vi "TAT_PLC_Data_read_BOLLEAN_I_O_SCREEN.vi"(7 "Enum":enum16{"Read", "Write"}(ring), 8 "error in (no error)":errorcluster, 10 "Array":bool[](array[boolean])) -> (0 "error out":errorcluster, 2 "Array 2":bool[](array[boolean]))   [LabVIEW 2017]
panel:
  # "INPUTS\t\t\nSR.NO\tPLC INPUT\tDESCRIPTION\tTO SOFTWARE MEMORY BIT\t\n1\tX0\tCYCLE START TOUCH BUTTON\tM0\t8192\n2\tX1\tCYCLE START TOUCH BUTTON\tM1\t8193\n3\tX2\tEMG STOP\tM2\t8194\n4\tX3\tRESET PB\tM3\t8195\n5\tX4\tPRESSURE SWITCH\tM4\t8196\n6\tX5\tSAFETY SENSOR\tM5\t8197\n7\tX6\tDOOR 1 \tM6\t8198\n8\tX7\tDOOR 2\tM7\t8199\n9\tX10\tSPARE\tM10\t8202\n10\tX11\tSHUTTLE OPEN CHECK SENSOR-X300\tM11\t8203\n11\tX12\tTHREAD LOCKER CYL COMPLETE\tM12\t8204\n12\tX13\tPUSHER HM RS\tM13\t8205\n13\tX14\tPUSHER END RS\tM14\t8206\n14\tX15\tUP DOWN CYL  HM RS\tM15\t8207\n15\tX16\tUP DOWN CYL END RS\tM16\t8208\n16\tX17\tPART CLAMP END RS\tM17\t8209\n17\tX20\t\tM20\t8212\n18\tX21\t\tM21\t8213\n19\tX22\t\tM22\t8214\n20\tX23\t\tM23\t8215\n21\tX24\t\tM24\t8216\n22\tX25\t\tM25\t8217\n\t\t\t\t\n\t\t\t\t\n\t\t\t\t\n\t\t\t\t\n\t\tOUTPUTS\t\t\nSR.NO\tPLC OUTPUT\tDESCRIPTION\tTO SOFTWARE MEMORY BIT\t\n1\tY0\tGREEN LAMP\tM30\t8222\n2\tY1\tRED LAMP\tM31\t8223\n3\tY2\tBUZZER\tM32\t8224\n4\tY3\tPART CLAMP SOL\tM33\t8225\n5\tY4\tTHREAD LOCKER ON\tM34\t8226\n6\tY5\tTHREAD LOCKER OFF\tM35\t8227\n7\tY6\tPUSHER FWD SOL\tM36\t8228\n8\tY7\tPUSHER REV SOL\tM37\t8229\n9\tY10\tUP DN CYL FWD SOL\tM38\t8230\n10\tY11\tUP DN CYL REV SOL\tM39\t8231\n11\tY12\t\tM40\t8232\n12\tY13\t\tM41\t8233\n13\tY14\t\tM42\t8234\n14\tY15\t\tM43\t8235\n15\tY16\t\tM44\t8236\n16\tY17\t\tM45\t8237\n17\tY20\t\tM46\t8238\n18\tY21\t\tM47\t8239"
  # "STATION 1\nand\nSTATION 2"
  # "CONTROL PROCESS TO  LABVIEW from PLC"
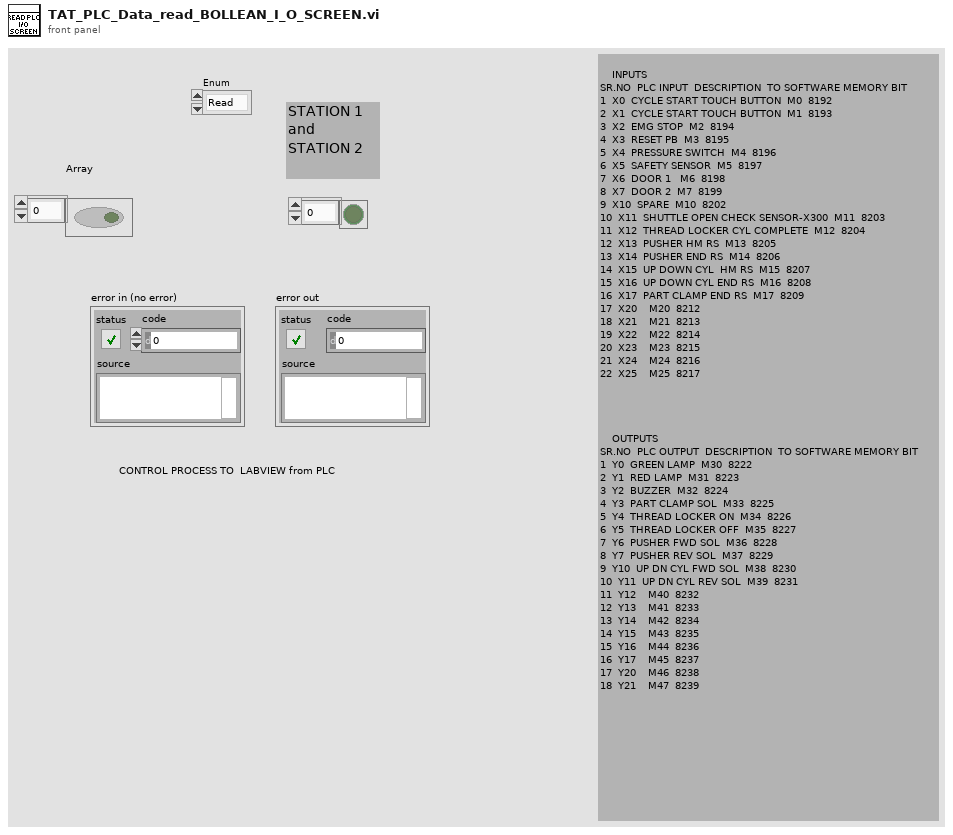
[diagram p1: front panel]
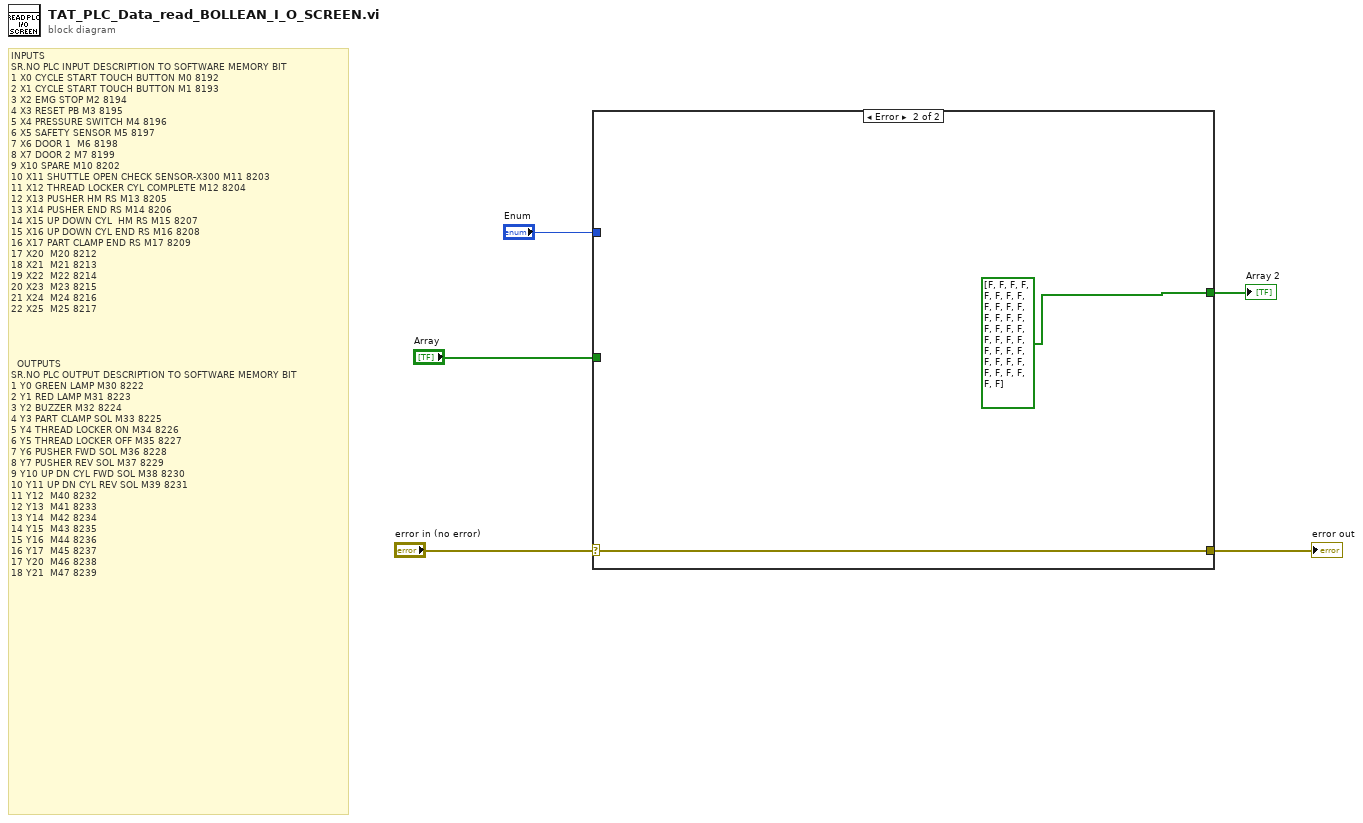
[diagram p0: block diagram]
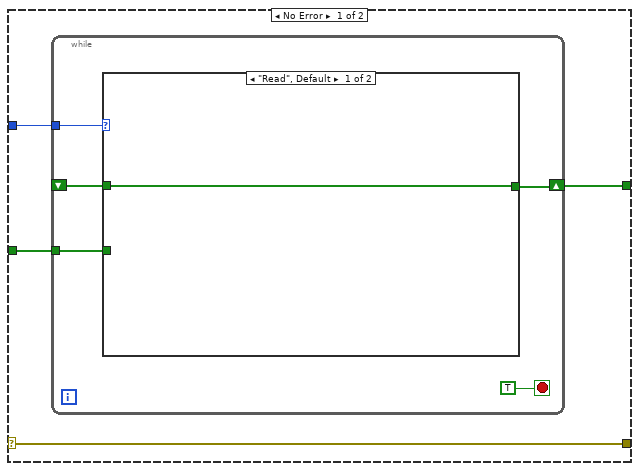
[diagram p2: hidden frame]
diagram:
  # "INPUTS\t\t\nSR.NO\tPLC INPUT\tDESCRIPTION\tTO SOFTWARE MEMORY BIT\t\n1\tX0\tCYCLE START TOUCH BUTTON\tM0\t8192\n2\tX1\tCYCLE START TOUCH BUTTON\tM1\t8193\n3\tX2\tEMG STOP\tM2\t8194\n4\tX3\tRESET PB\tM3\t8195\n5\tX4\tPRESSURE SWITCH\tM4\t8196\n6\tX5\tSAFETY SENSOR\tM5\t8197\n7\tX6\tDOOR 1 \tM6\t8198\n8\tX7\tDOOR 2\tM7\t8199\n9\tX10\tSPARE\tM10\t8202\n10\tX11\tSHUTTLE OPEN CHECK SENSOR-X300\tM11\t8203\n11\tX12\tTHREAD LOCKER CYL COMPLETE\tM12\t8204\n12\tX13\tPUSHER HM RS\tM13\t8205\n13\tX14\tPUSHER END RS\tM14\t8206\n14\tX15\tUP DOWN CYL  HM RS\tM15\t8207\n15\tX16\tUP DOWN CYL END RS\tM16\t8208\n16\tX17\tPART CLAMP END RS\tM17\t8209\n17\tX20\t\tM20\t8212\n18\tX21\t\tM21\t8213\n19\tX22\t\tM22\t8214\n20\tX23\t\tM23\t8215\n21\tX24\t\tM24\t8216\n22\tX25\t\tM25\t8217\n\t\t\t\t\n\t\t\t\t\n\t\t\t\t\n\t\t\t\t\n\t\tOUTPUTS\t\t\nSR.NO\tPLC OUTPUT\tDESCRIPTION\tTO SOFTWARE MEMORY BIT\t\n1\tY0\tGREEN LAMP\tM30\t8222\n2\tY1\tRED LAMP\tM31\t8223\n3\tY2\tBUZZER\tM32\t8224\n4\tY3\tPART CLAMP SOL\tM33\t8225\n5\tY4\tTHREAD LOCKER ON\tM34\t8226\n6\tY5\tTHREAD LOCKER OFF\tM35\t8227\n7\tY6\tPUSHER FWD SOL\tM36\t8228\n8\tY7\tPUSHER REV SOL\tM37\t8229\n9\tY10\tUP DN CYL FWD SOL\tM38\t8230\n10\tY11\tUP DN CYL REV SOL\tM39\t8231\n11\tY12\t\tM40\t8232\n12\tY13\t\tM41\t8233\n13\tY14\t\tM42\t8234\n14\tY15\t\tM43\t8235\n15\tY16\t\tM44\t8236\n16\tY17\t\tM45\t8237\n17\tY20\t\tM46\t8238\n18\tY21\t\tM47\t8239"
  n1 = case shown="Error" "error in (no error)" {
    selector: "error in (no error)" -> [w6 w18]
    tunnel: [w6 w18] -> w5
    tunnel: "Enum" -> [w9 _]
    tunnel: "Array" -> [w8 _]
    tunnel: [w7 bool[] [FALSE, FALSE, FALSE, FALSE, FALSE, FALSE, FALSE, FALSE, FALSE, FALSE, FALSE, FALSE, FALSE, FALSE, FALSE, FALSE, FALSE, FALSE, FALSE, FALSE, FALSE, FALSE, FALSE, FALSE, FALSE, FALSE, FALSE, FALSE, FALSE, FALSE, FALSE, FALSE, FALSE, FALSE, FALSE, FALSE, FALSE, FALSE]] -> w1
    frame No Error {
      n2 = while {
        tunnel: w9 -> [w13]
        shift-right: [w10] -> w7
        shift-left: _ -> [w11]
        tunnel: w8 -> [w12]
        stop <- TRUE stop-if-true
        n3 = case shown="\"Read\", Default" w13 {
          tunnel: w12 -> [_ w16]
          tunnel: [w15 w16] -> w10
          tunnel: w11 -> [w15 _]
          frame "Read", Default {
          }
          frame "Write" {
          }
        }
      }
    }
    frame Error {
    }
  }
  "error out" <- w5
  "Array 2" <- w1
